vi "HSE Logger Custom Probe - DEBUG (Error).vi"(11 "error out":errorcluster) -> (2 "Value String":string, 3 "Boolean":bool)   [LabVIEW 2016]
uses:
  HSE-Logger/hse-logger.lvlib
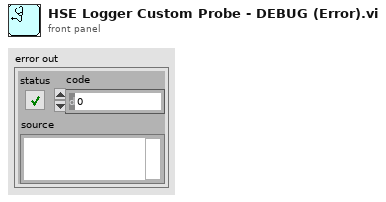
[diagram p1: front panel]
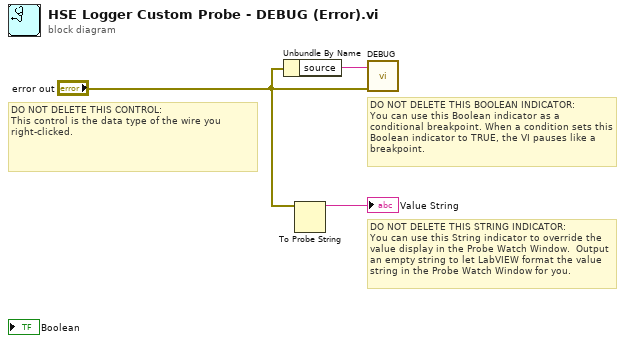
[diagram p0: block diagram]
diagram:
  # "DO NOT DELETE THIS STRING INDICATOR: \nYou can use this String indicator to override the value display in the Probe Watch Window.  Output an empty string to let LabVIEW format the value string in the Probe Watch Window for you."
  # "DO NOT DELETE THIS BOOLEAN INDICATOR: \nYou can use this Boolean indicator as a conditional breakpoint. When a condition sets this Boolean indicator to TRUE, the VI pauses like a breakpoint."
  # "DO NOT DELETE THIS CONTROL: \nThis control is the data type of the wire you right-clicked."
  n1 = Unbundle By Name("error out") -> ("source"=w2:string)
  n2 = To Probe String(7:"error out") -> (3:→"Value String":string)  [unwired: 2 in, 1 out]
  n3 = call "DEBUG.vi"("Message"=w2, "error in"="error out") -> ()  [unwired: 9 in, 1 out]
